vi "MyG#Class_Create.vi"(0 "reference in":refnum<class "MyG#Class.lvclass">, 1 "MyAttribute":dbl, 5 "error in (no error)":errorcluster) -> (14 "reference out":refnum<class "MyG#Class.lvclass">, 19 "error out":errorcluster)   [LabVIEW 2020, in "MyG#Class.lvclass"]
doc: "Constructor."
uses:
  MyG#Class.lvclass
  C:/ProjectGSharpDevelopment_2020-3/gsharp/VIPM/Files/vi.lib/addons/_AddQ/G#Object/G#Object.lvclass
  vi.lib/addons/_AddQ/G#Object/G#Object.lvclass
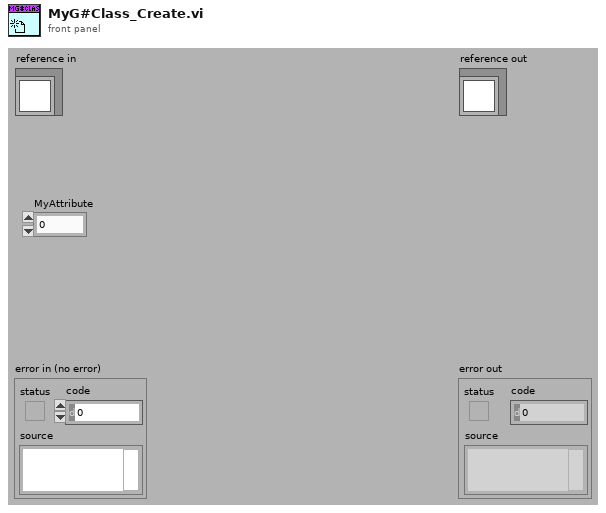
[diagram p1: front panel]
types:
  T1 = typedef "MyG#Class.lvclass/ObjectAttributesRef.ctl" = refnum<data-value>
  T2 = typedef "MyG#Class.lvclass/ObjectAttributes.ctl" = cluster{"MyAttribute":dbl}
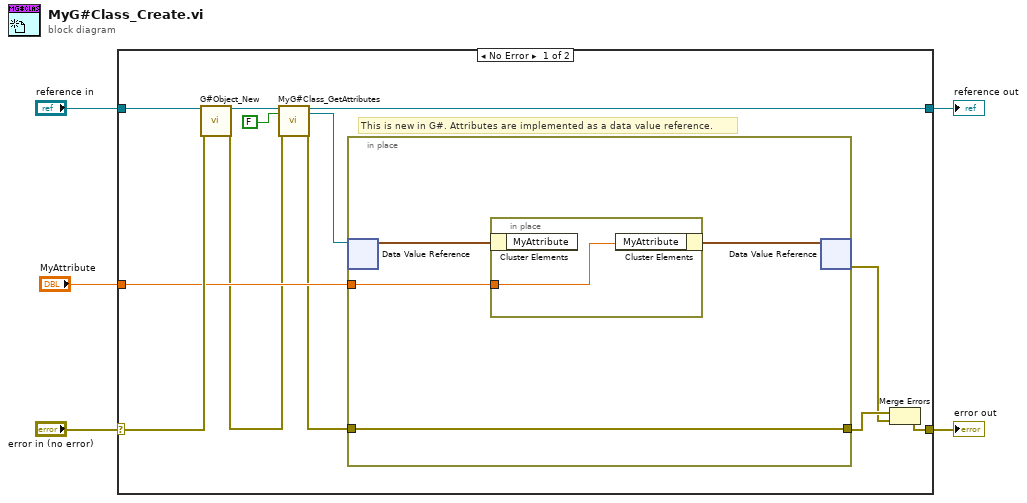
[diagram p0: block diagram]
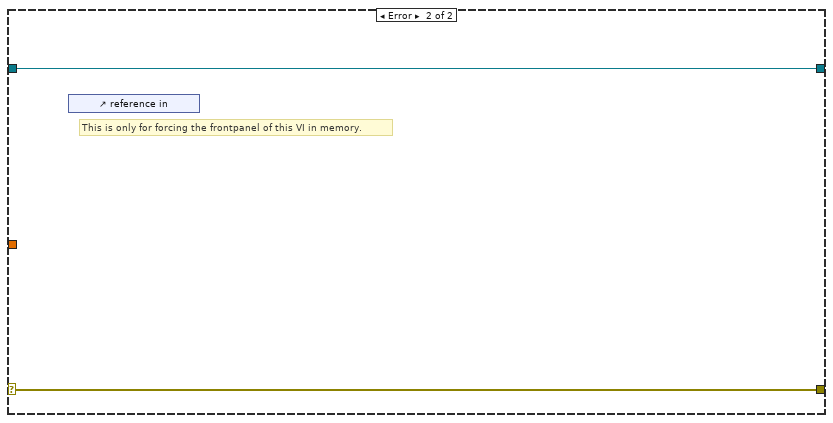
[diagram p2: hidden frame]
diagram:
  n1 = case shown="No Error" "error in (no error)" {
    selector: "error in (no error)" -> [w16 w24]
    tunnel: [w15 w24] -> w4
    tunnel: [w10 w23] -> w2
    tunnel: "reference in" -> [w17 w23]
    tunnel: "MyAttribute" -> [w12 _]
    frame No Error {
      # "This is new in G#. Attributes are implemented as a data value reference."
      n2 = call "G#Object_New.vi"("reference in"=w17, "error in (no error)"=w16) -> ("reference out"=w11:refnum<class "MyG#Class.lvclass">, "error out"=w9:errorcluster)  [unwired: 15 in, 1 out]
      n3 = call "MyG#Class_GetAttributes.vi"("reference in"=w11, "return data? (T)"=FALSE, "error in (no error)"=w9) -> ("reference out"=w10:refnum<class "MyG#Class.lvclass">, "attributes ref"=w7:T1, "error out"=w8:errorcluster)  [unwired: 13 in, 1 out]
      n4 = in-place {
        in-place-border: w8 -> [w19]
        in-place-border: [w19] -> w14
        in-place-border: w12 -> [w18]
        n5 = in-place-dvr #1(w7) -> (w20:T2)  [unwired: 1 out]
        n6 = in-place {
          in-place-border: w18 -> [w22]
          n7 = in-place-cluster #2(w20) -> ()  [unwired: 1 out]
          n8 = in-place-cluster #2("MyAttribute"=w22) -> (w21:T2)
        }
        n9 = in-place-dvr #1(w21) -> (w13:errorcluster)  [unwired: 1 out]
      }
      n10 = Merge Errors(w14, w13) -> (w15:errorcluster)
    }
    frame Error {
      # "This is only for forcing the frontpanel of this VI in memory."
      n11 = control-ref of="reference in"() -> ()  [unwired: 1 out]
    }
  }
  "error out" <- w4
  "reference out" <- w2
